vi "Configure Sine.vi"(3 "phase(deg)":dbl, 4 "amplitude":dbl=1.0, 5 "frequency":dbl=1000.0) -> (0 "error out":errorcluster, 1 "refOut":u32)   [LabVIEW 2021]
uses:
  <vilib>/addons/_NISVFA/_Generation/Signal Generation/SV Signal/SV Signal.lvclass
  <vilib>/addons/_NISVFA/_Generation/Signal Generation/SV Sinusoid/SV Sinusoid.lvclass
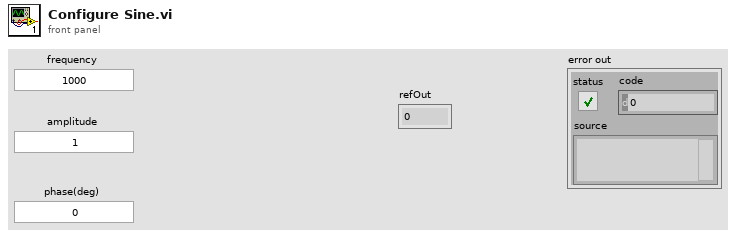
[diagram p1: front panel]
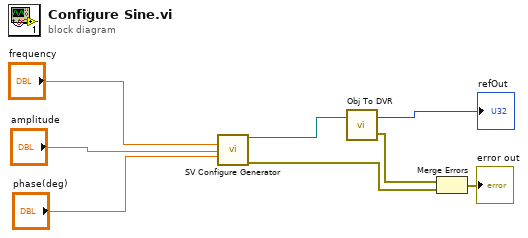
[diagram p0: block diagram]
diagram:
  n1 = call-poly <vilib>:"SV Configure Generator.vi"("frequency (Hz)"="frequency", "amplitude"="amplitude", "phase (deg)"="phase(deg)") -> ("signal configuration"=w5:refnum<class "SV Sinusoid.lvclass">, "error out"=w2:errorcluster)  [unwired: 11 in]
  n2 = call "Obj To DVR.vi"("signal configuration"=w5) -> ("error_out"=w3:errorcluster, "dataValueReference"=→"refOut":u32)  [unwired: 1 in]
  n3 = Merge Errors(w3, w2) -> (→"error out":errorcluster)
